vi "FlowCalc.vi"(9 "Individual Channel Cluster":T1, 11 "Flow":fxp<+/-,24,-4>) -> (0 "Flow - No Operations":bool, 1 "Flow - Warning":bool, 3 "Flow Rate":dbl)   [LabVIEW 2016]
panel:
  out "Channel":string
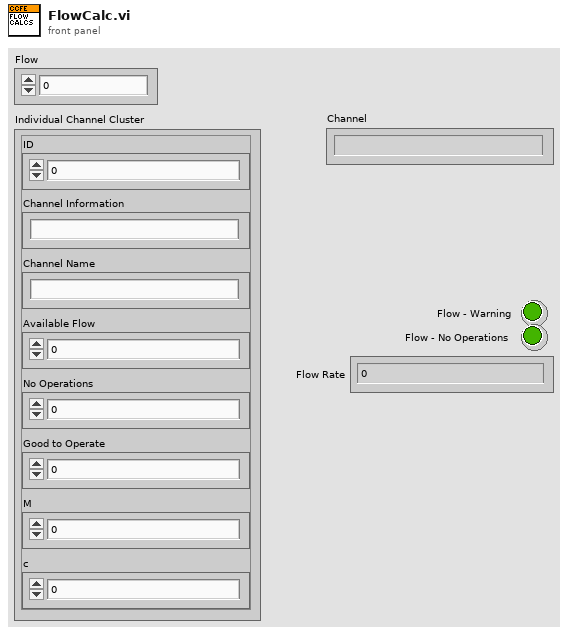
[diagram p1: front panel]
types:
  T1 = cluster{"ID":i32, "Channel Information":string, "Channel Name":string, "Available Flow":dbl, "No Operations":dbl, "Good to Operate":dbl, "M":dbl, "c":dbl}
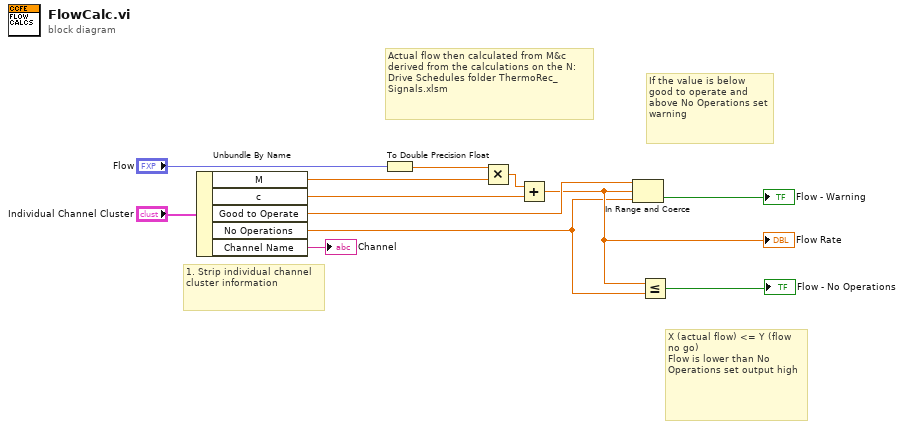
[diagram p0: block diagram]
diagram:
  # "X (actual flow) <= Y (flow no go)\nFlow is lower than No Operations set output high"
  # "If the value is below good to operate and above No Operations set warning"
  # "Actual flow then calculated from M&c derived from the calculations on the N: Drive Schedules folder ThermoRec_Signals.xlsm"
  # "1. Strip individual channel cluster information"
  n1 = Unbundle By Name("Individual Channel Cluster") -> ("M"=w9:dbl, "c"=w8:dbl, "Good to Operate"=w7:dbl, "No Operations"=w5:dbl, "Channel Name"=→"Channel":string)
  n2 = To Double Precision Float(number="Flow") -> (double precision float=w12:dbl)
  n3 = Multiply(x=w12, y=w9) -> (x*y=w11:dbl)
  n4 = Add(x=w11, y=w8) -> (x+y=w6:dbl)
  "Flow Rate" <- w6
  n5 = In Range and Coerce(upper limit=w7, x=w6, lower limit=w5) -> (In Range?=→"Flow - Warning":bool)  [unwired: 1 out]
  n6 = Less Or Equal?(x=w6, y=w5) -> (x <= y?=→"Flow - No Operations":bool)
